vi "DT_Find Next Triangulation_Update Candidate.vi"(9 "Data In":T1, 10 "Triangles In":i32[][](array[numeric]), 11 "Points In":cluster{"x":dbl, "y":dbl, "index":i32}[](array[cluster])) -> (0 "error":i32, 1 "Data Out":T1, 2 "Triangles Out":i32[][](array[numeric]), 3 "Points Out":cluster{"x":dbl, "y":dbl, "index":i32}[](array[cluster]))   [LabVIEW 2017, in "NI_AAL_Geometry.lvlib"]
uses:
  <vilib>/Analysis/NI_AAL_Geometry.lvlib
  <vilib>/Analysis/geometry.llb/DT_Find Next Triangulation_Data.ctl
  <vilib>/Analysis/geometry.llb/DT_Triangle Manager_Get Oppo Point_in Ghost.vi
  <vilib>/Analysis/geometry.llb/DT_Triangle Manager_Get Global Point Index.vi
  <vilib>/Analysis/geometry.llb/DT_Triangle Manager_Get Adj_by Edge.vi
  <vilib>/Analysis/geometry.llb/DT_Triangle Manager_Get Local Point Index.vi
  <vilib>/Analysis/geometry.llb/DT_Triangle Manager_Get Oppo Point.vi
  <vilib>/Analysis/geometry.llb/DT_Triangle Manager_Get Ghost Point.vi
  <vilib>/Analysis/geometry.llb/DT_Triangle Manager_Get Adj_by Point.vi
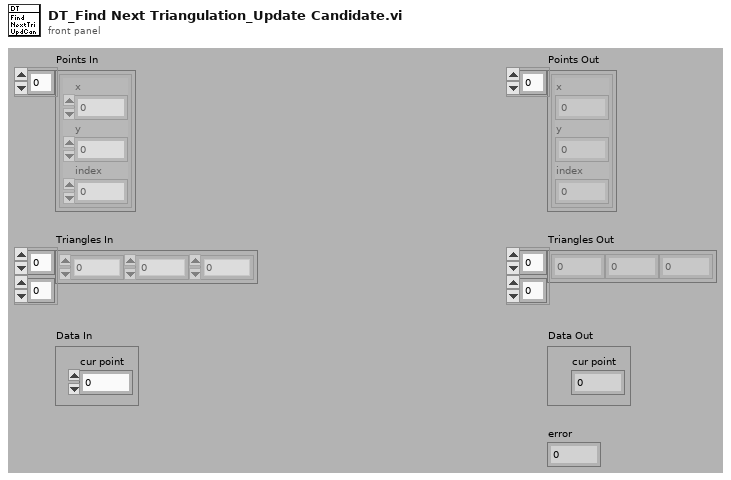
[diagram p1: front panel]
types:
  T1 = typedef "NI_AAL_Geometry.lvlib/DT_Find Next Triangulation_Data.ctl" = cluster{"cur point":i32, "cur triangle":i32, "cur local idx":i32, "base point":i32, "base triangle":i32, "base local idx":i32, "Candidate Triangles":i32[], "Candidate Point Idx":i32[]}
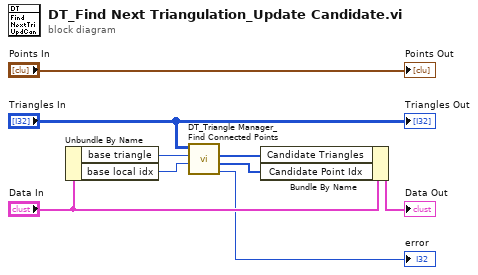
[diagram p0: block diagram]
diagram:
  n1 = Unbundle By Name("Data In") -> ("base triangle"=w8:i32, "base local idx"=w7:i32)
  n2 = call <vilib>:"DT_Triangle Manager_Find Connected Points.vi"("base point idx"=w7, "triangle"=w8, "Triangles"="Triangles In") -> ("error"=→"error":i32, "Connected Point Idx"=w5:i32[], "Connected Triangles"=w6:i32[])  [unwired: 6 out]
  n3 = Bundle By Name(cluster="Data In", "Candidate Triangles"=w6, "Candidate Point Idx"=w5) -> (→"Data Out":T1)
  "Points Out" <- "Points In"
  "Triangles Out" <- "Triangles In"
